vi "SetPower.vi"(8 "error in (no error)":errorcluster, 10 "MotorPower Terminal":dbl(slide) scale=-1.0..1.0, 11 "DriveMotors in":refnum<class "DriveMotors.lvclass">) -> (0 "error out":errorcluster, 3 "DriveMotors out":refnum<class "DriveMotors.lvclass">)   [LabVIEW 2013, in "DriveMotors.lvclass"]
uses:
  DriveMotors.lvclass
  DriveMotors.lvclass/DriveMotors.ctl
  Utilities/Event/Event.lvclass
  EventMgr/EventMgr.lvclass
  <vilib>/addons/control/pid/pid.llb/PID (DBL).vi
  Robot Global Data.vi
  <vilib>/addons/control/pid/NI_PID_pid.lvlib
panel:
  in  "dt (s)":dbl=-1.0 format="%.3f"
  in  "MotorPower Virtual":dbl(slide) step=0.05 scale=-1.0..1.0
  in  "Use Virtual":bool
  out "PID Power":dbl
  in  "MaxGain":dbl=0.5 min=0.0 max=1.0 step=0.001
  out "output":dbl format="%.2f"
  out "Rate (PV)":dbl
  out "Rate (SP)":dbl
  in  "PID gains":T1={"proportional gain (Kc)"=0.01, "integral time (Ti, min)"=0.0, "derivative time (Td, min)"=0.0} {"derivative time (Td, min)" format="%.3f"; "integral time (Ti, min)" format="%.3f"; "proportional gain (Kc)" format="%.3f"}
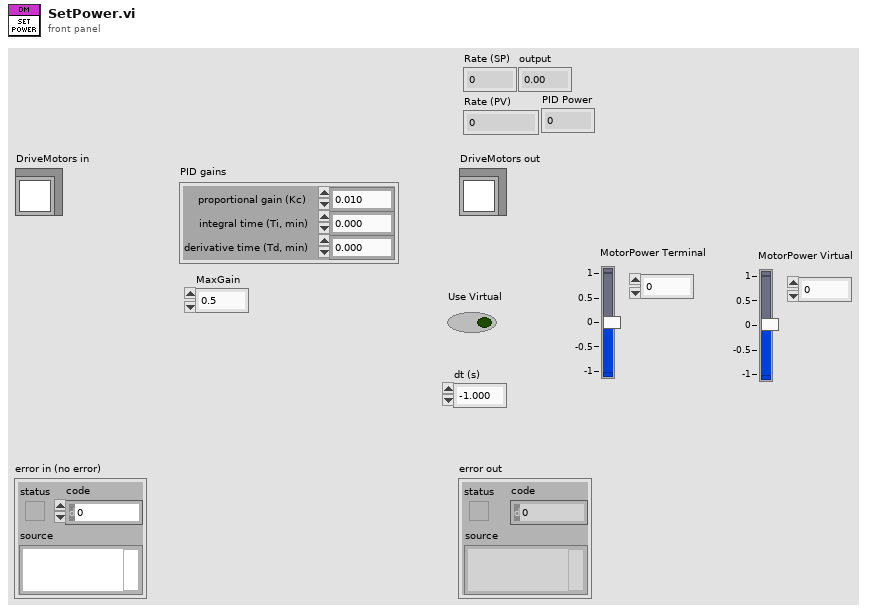
[diagram p1: front panel]
types:
  T1 = cluster{"proportional gain (Kc)":dbl, "integral time (Ti, min)":dbl, "derivative time (Td, min)":dbl}
  T2 = typedef "WPI_MotorControlDeviceRef.ctl" = cluster{"DeviceStatus":errorcluster, "Type":enum16{"PWM", "CAN"}, "PWM":cluster{"Digital Module":T3, "PWM Channel":T4, "DeadBand":T5}, "CAN":cluster{"Device Number":u8, "Control Mode":T6, "Semaphore":T7, "Max Vout":dbl}, "Invert":bool, "TransformRef":T8, "InvTransformRef":T8}
  T3 = typedef "FPGA_TypedefDigitalModule.ctl" = enum16{"Digital Module 1", "Digital Module 2"}
  T4 = typedef "FPGA_DIOPWMChannel.ctl" = enum8{"PWM 1", "PWM 2", "PWM 3", "PWM 4", "PWM 5", "PWM 6", "PWM 7", "PWM 8", "PWM 9", "PWM 10", "Invalid"}
  T5 = typedef "WPI_PWMDeadband.ctl" = cluster{"Name":string, "maxPositivePwm":i32, "minPositivePwm":i32, "centerPwm":i32, "maxNegativePwm":i32, "minNegativePwm":i32, "angularRange":u16}
  T6 = typedef "WPI_CANJaguar_ControlMode.ctl" = enum8{"Percent VBus", "Current", "Speed", "Position", "Voltage"}
  T7 = typedef "Semaphore RefNum" = refnum<k1>
  T8 = typedef "WPI_PWMTransform_ConPane.ctl" = refnum<vi>
  T9 = typedef "WPI_EncoderDevRef.ctl" = cluster{"DevStatus":errorcluster, "EncoderIndex":T10, "CounterIndex":T11, "DistancePerCount":dbl, "Decoding Type":T12}
  T10 = typedef "FPGA_EncoderIdx.ctl" = enum8{"Enc 0", "Enc 1", "Enc 2", "Enc 3", "Invalid"}
  T11 = typedef "FPGA_CounterCtrSystemIndex.ctl" = enum8{"Ctr 0", "Ctr 1", "Ctr 2", "Ctr 3", "Ctr 4", "Ctr 5", "Ctr 6", "Ctr 7", "Invalid"}
  T12 = typedef "WPI_EncoderType.ctl" = enum16{"1x", "2x", "4x"}
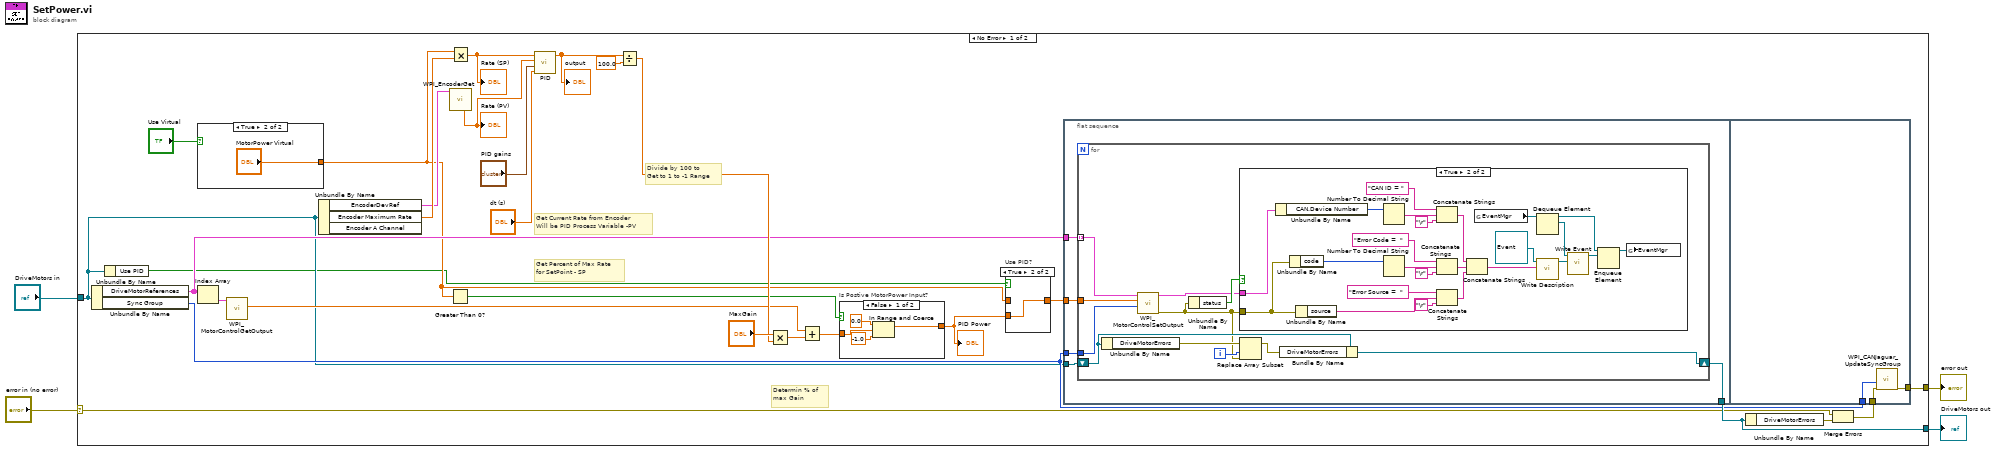
[diagram p0: block diagram]
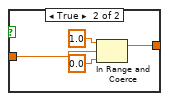
[diagram p2: hidden frame]
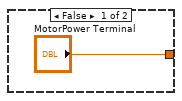
[diagram p3: hidden frame]
diagram:
  n1 = case shown="No Error" "error in (no error)" {
    selector: "error in (no error)" -> [w29 w89]
    tunnel: [w32 w89] -> w3
    tunnel: [w31 w88] -> w1
    tunnel: "DriveMotors in" -> [w6 w88]
    frame No Error {
      # "Determin % of \nmax Gain"
      # "Divide by 100 to \nGet to 1 to -1 Range"
      # "Get Percent of Max Rate\nfor SetPoint - SP"
      # "Get Current Rate from Encoder\nWill be PID Process Variable -PV"
      n2 = Unbundle By Name(w6) -> ("DriveMotorReferences"=w17:T2[], "Sync Group"=w27:u8)
      n3 = Unbundle By Name(w6) -> ("Use PID"=w5:bool)
      n4 = case shown="True" "Use Virtual" {
        tunnel: ["MotorPower Terminal" "MotorPower Virtual"] -> w11
        frame False {
        }
        frame True {
        }
      }
      n5 = Index Array(array=w17) -> (element=w16:T2)  [unwired: 1 in]
      n6 = call <vilib>:"WPI_MotorControlGetOutput.vi"("MotorControlDevRef"=w16) -> ("Output"=w14:dbl)  [unwired: 8 in, 2 out]
      n7 = Unbundle By Name(w6) -> ("EncoderDevRef"=w23:T9, "Encoder Maximum Rate"=w25:dbl)  [unwired: 1 out]
      n8 = Greater Than 0?(x=w11) -> (x > 0?=w8:bool)
      n9 = Multiply(x=w11, y=w25) -> (x*y=w24:dbl)
      "Rate (SP)" <- w24
      n10 = call <vilib>:"WPI_EncoderGet.vi"("EncoderDevRef"=w23) -> ("Rate"=w22:dbl)  [unwired: 1 in, 9 out]
      "Rate (PV)" <- w22
      n11 = call-poly <vilib>:"PID.vi"("dt (s)"="dt (s)", "PID gains"="PID gains", "process variable"=w22, "setpoint"=w24) -> ("output"=w21:dbl)  [unwired: 6 in, 1 out]
      "output" <- w21
      n12 = Divide(x=w21, y=100.0) -> (x/y=w18:dbl)
      n13 = Multiply(x="MaxGain", y=w18) -> (x*y=w15:dbl)
      n14 = Add(x=w14, y=w15) -> (x+y=w10:dbl)
      n15 = case "Is Postive MotorPower Input?" shown="False" w8 {
        tunnel: w10 -> [w36 w40]
        tunnel: [w33 w37] -> w9
        frame False {
          n16 = In Range and Coerce(upper limit=0.0, x=w36, lower limit=-1.0) -> (coerced(x)=w33:dbl)  [unwired: 1 out]
        }
        frame True {
          n17 = In Range and Coerce(upper limit=1.0, x=w40, lower limit=0.0) -> (coerced(x)=w37:dbl)  [unwired: 1 out]
        }
      }
      "PID Power" <- w9
      n18 = case "Use PID?" shown="True" w5 {
        tunnel: w11 -> [w43 _]
        tunnel: [w43 w44] -> w13
        tunnel: w9 -> [_ w44]
        frame False {
        }
        frame True {
        }
      }
      n19 = flat-sequence {
        tunnel: w17 -> [w49]
        tunnel: w27 -> [w45]
        tunnel: w13 -> [w48]
        tunnel: w6 -> [w46]
        tunnel: [w47] -> w31
        tunnel: w27 -> [w87]
        tunnel: w28 -> [w86]
        tunnel: [w85] -> w32
        frame #0 {
          n20 = for {
            tunnel: w49 -> [w60] mode=indexing
            tunnel: w48 -> [w59]
            shift-right: [w56] -> w47
            shift-left: w46 -> [w54]
            tunnel: w45 -> [w53]
            i -> [w58]
            n21 = Unbundle By Name(w54) -> ("DriveMotorErrors"=w55:errorcluster[])
            n22 = call <vilib>:"WPI_MotorControlSetOutput.vi"("Sync Group"=w53, "Output"=w59, "MotorControlDevRef"=w60) -> ("error out"=w50:errorcluster, "MotorControlDevRef"=w51:T2)  [unwired: 6 in, 1 out]
            n23 = Unbundle By Name(w50) -> ("status"=w52:bool)
            n24 = case shown="True" w52 {
              tunnel: w51 -> [_ w83]
              tunnel: w50 -> [_ w67]
              frame False {
              }
              frame True {
                n25 = Unbundle By Name(w83) -> ("CAN.Device Number"=w82:u8)
                n26 = Unbundle By Name(w67) -> ("code"=w66:i32)
                n27 = Unbundle By Name(w67) -> ("source"=w70:string)
                n28 = Number To Decimal String(number=w82) -> (decimal integer string=w81:string)  [unwired: 1 in]
                n29 = Number To Decimal String(number=w66) -> (decimal integer string=w74:string)  [unwired: 1 in]
                n30 = Concatenate Strings("CAN ID = ", w81, "\r") -> (w79:string)
                n31 = Concatenate Strings("Error Code =  ", w74, "\r") -> (w72:string)
                n32 = Concatenate Strings("Error Source =  ", w70, "\r") -> (w68:string)
                n33 = Concatenate Strings(w79, w72, w68) -> (w77:string)
                n34 = global read "Robot Global Data.vi" "EventMgr"() -> (w65:refnum<queue>)
                n35 = Dequeue Element(queue=w65) -> (queue out=w62:refnum<queue>, element=w64:refnum<class "EventMgr.lvclass">)  [unwired: 2 in, 2 out]
                n36 = call-dynamic "Write Description.vi"("Description"=w77, "Event in"=refnum<class "Event.lvclass"> refnum ("Event.lvclass")) -> ("Event out"=w76:refnum<class "Event.lvclass">)  [unwired: 8 in, 1 out]
                n37 = call-dynamic "Write Event.vi"("Event"=w76, "EventMgr in"=w64) -> ("EventMgr out"=w63:refnum<class "EventMgr.lvclass">)  [unwired: 8 in, 1 out]
                n38 = Enqueue Element(queue=w62, element=w63) -> (queue out=w61:refnum<queue>)  [unwired: 2 in, 2 out]
                n39 = global write "Robot Global Data.vi" "EventMgr"(w61) -> ()
              }
            }
            n40 = Replace Array Subset(array=w55, new element=w50, index=w58) -> (w57:errorcluster[])
            n41 = Bundle By Name(cluster=w54, "DriveMotorErrors"=w57) -> (w56:refnum<class "DriveMotors.lvclass">)
          }
        }
        frame #1 {
          n42 = call <vilib>:"WPI_CANJaguar_UpdateSyncGroup.vi"("error in (no error)"=w86, "Sync Group"=w87) -> ("error out"=w85:errorcluster)  [unwired: 9 in]
        }
      }
      n43 = Unbundle By Name(w31) -> ("DriveMotorErrors"=w30:errorcluster[])
      n44 = Merge Errors(w29, w30) -> (w28:errorcluster)
    }
    frame Error {
    }
  }
  "error out" <- w3
  "DriveMotors out" <- w1
